vi "JKISM-Reuse Module.vi"(7 "Name(\"\" to use uuid)":string="Event JKISM") -> ()   [LabVIEW 2014]
uses:
  user.lib/_NEVSTOP/JKI State Machine++/_Support/JKISMQ/_Obtain JKISMQ.vi
  user.lib/_NEVSTOP/JKI State Machine++/_Support/FGV-BroadcastRegistry/Cache-Broadcast Registry Search Result.vi
  user.lib/_NEVSTOP/JKI State Machine++/AdvanceAPI/JKISM++ Register Status Change.vi
  user.lib/_NEVSTOP/JKI State Machine++/AdvanceAPI/JKISM++ Unregister Status Change.vi
  user.lib/_NEVSTOP/JKI State Machine++/_Support/JKISMQ/_Create Resp Queue.vi
  user.lib/_NEVSTOP/JKI State Machine++/_Support/JKISMQ/_Unlock JKISMQ.vi
  user.lib/_NEVSTOP/JKI State Machine++/_Support/JKISMQ/_Lock State JKISMQ.vi
  user.lib/_NEVSTOP/JKI State Machine++/_Support/JKISMQ/_Release JKISMQ.vi
  user.lib/_NEVSTOP/JKI State Machine++/AdvanceAPI/JKISM++ Make String Arguments Safe.vi
  user.lib/_NEVSTOP/JKI State Machine++/_Support/JKISMQ/_Input Name to JKISM Mode.vi
  user.lib/_NEVSTOP/JKI State Machine++/Utility/uuid.vi
  user.lib/_NEVSTOP/JKI State Machine++/_Support/KeyWords.vi
  user.lib/_NEVSTOP/JKI State Machine++/_Support/FGV-BroadcastRegistry/global-JKISMQ FGV Change Flag.vi
  user.lib/_NEVSTOP/JKI State Machine++/_Support/JKISMQ/_JKISMQFGV.vi
  user.lib/_NEVSTOP/JKI State Machine++/_Support/GlobalEvent/FGV-GlobalEventRef.vi
  user.lib/_NEVSTOP/JKI State Machine++/_Support/JKISMQ/_Dequeue JKISMQ.vi
  user.lib/_NEVSTOP/JKI State Machine++/_Support/JKISMQ/_Enqueue JKISMQ.vi
  user.lib/_NEVSTOP/JKI State Machine++/_Support/FGV-BroadcastRegistry/global-Broadcast Cache Change Flag.vi
  user.lib/_NEVSTOP/JKI State Machine++/_Support/FGV-BroadcastRegistry/FGV-BroadcastRegistry.vi
  user.lib/_NEVSTOP/JKI State Machine++/JKI State Machine++.lvlib
panel:
  in  "Stop":bool
  in  "Start":bool
  out "publish status":bool
  out "Random":dbl
  in  "Level":dbl=0.5 format="%#_13g"
  out "State History":string
  # ">"
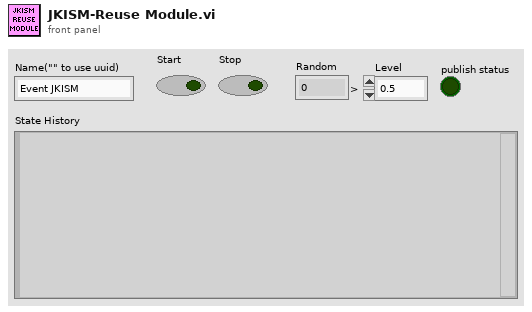
[diagram p1: front panel]
types:
  T1 = enum32{"Invalid", "Standard", "Closed", "Hidden", "Minimized", "Maximized"}
  T2 = enum32{"invalid app kind", "Development System", "Run Time System", "Student Edition", "Embedded LabVIEW", "Evaluation", "Custom"}
  T3 = cluster{"Core":cluster{"Current VI Reference":refnum<vi>, "Close Panel on Exit?":bool}, "Your Boolean data":bool, "Your string data":string}
  T4 = cluster{"Current VI Reference":refnum<vi>, "Close Panel on Exit?":bool}
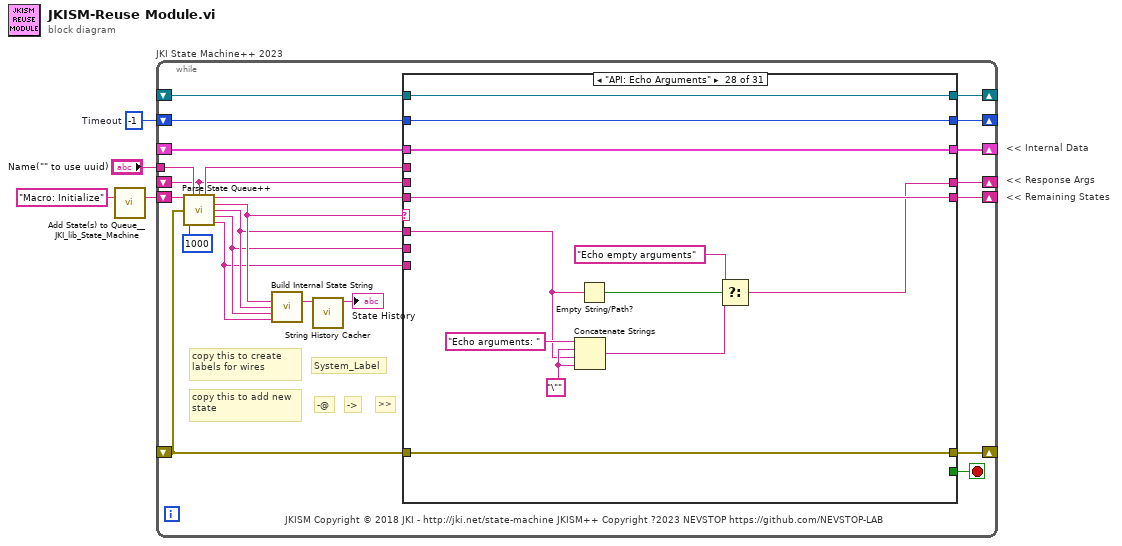
[diagram p0: block diagram]
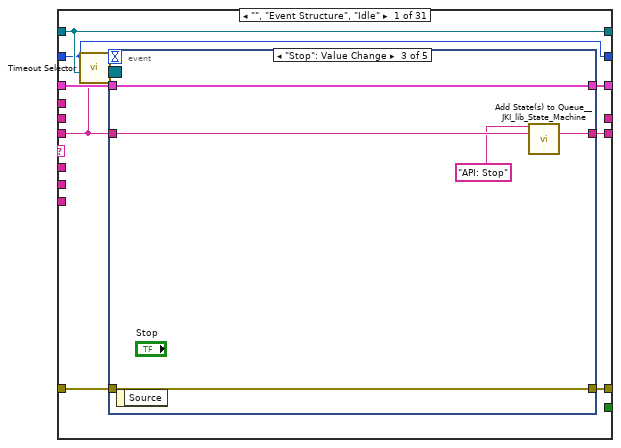
[diagram p2: hidden frame]
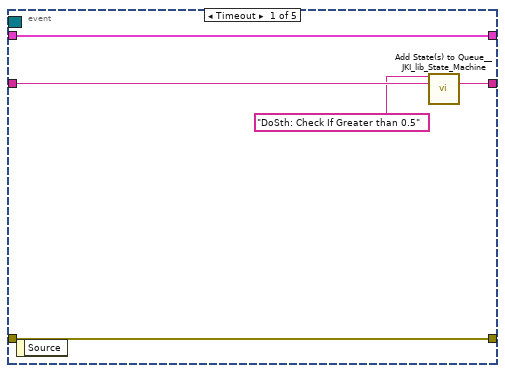
[diagram p3: hidden frame]
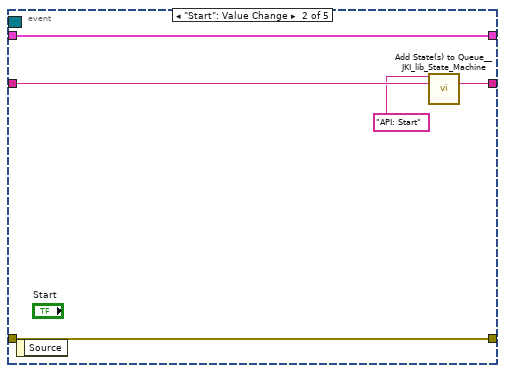
[diagram p4: hidden frame]
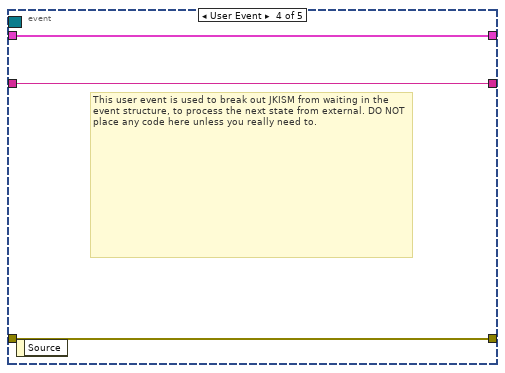
[diagram p5: hidden frame]
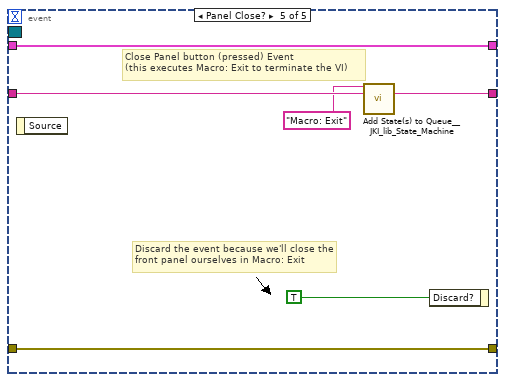
[diagram p6: hidden frame]
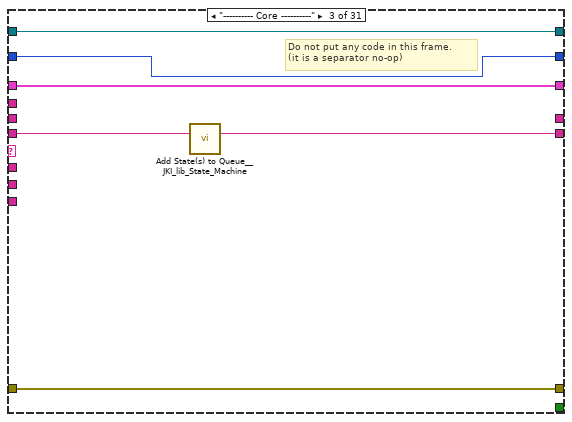
[diagram p8: hidden frame]
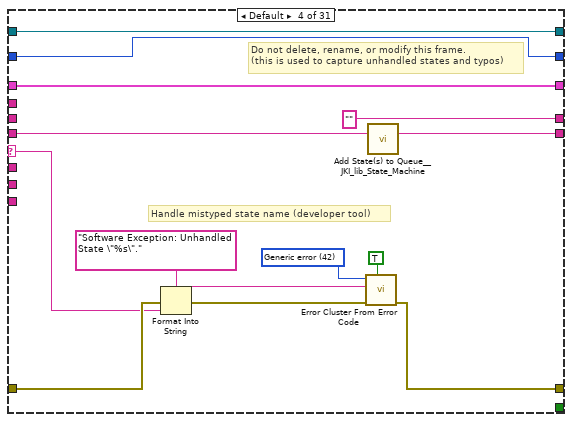
[diagram p9: hidden frame]
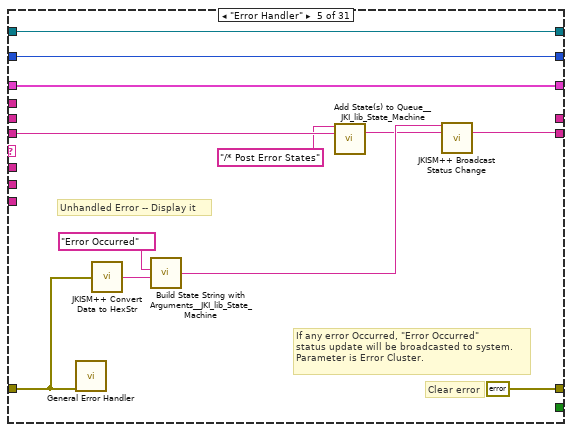
[diagram p10: hidden frame]
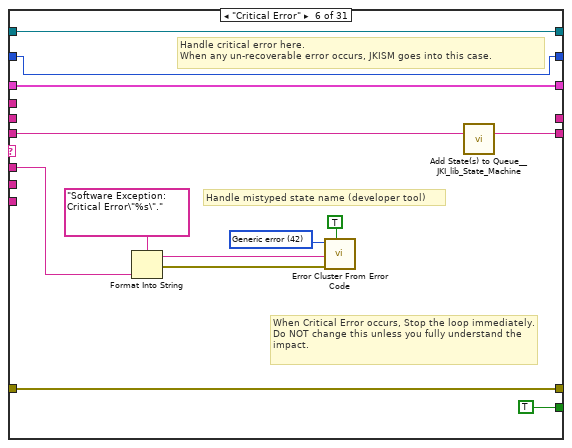
[diagram p11: hidden frame]
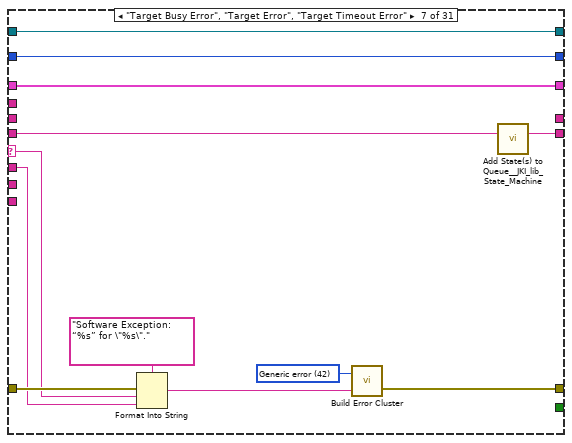
[diagram p12: hidden frame]
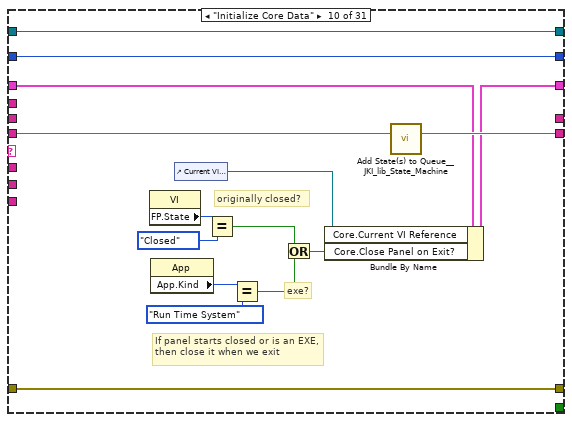
[diagram p15: hidden frame]
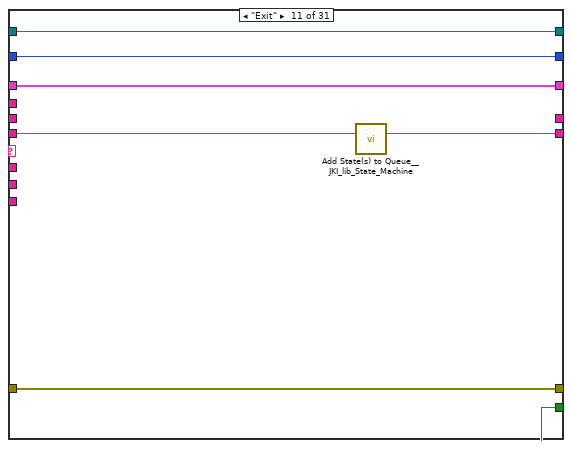
[diagram p16: hidden frame]
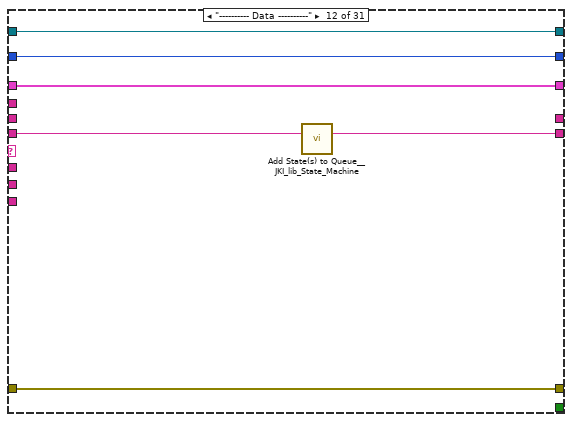
[diagram p17: hidden frame]
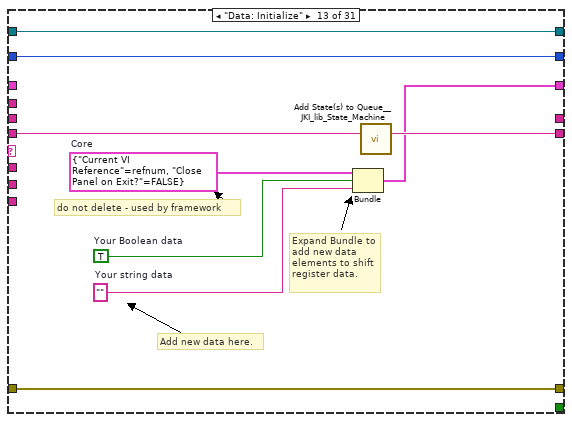
[diagram p18: hidden frame]
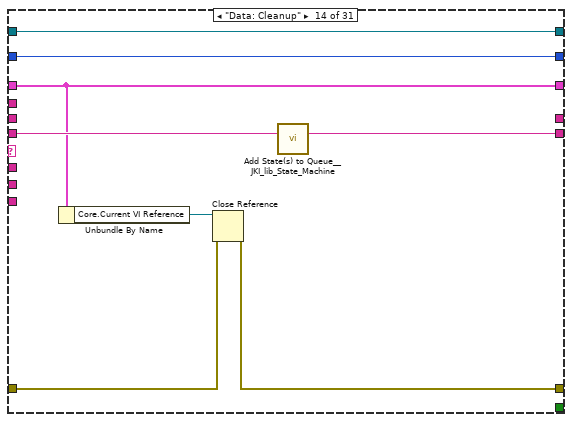
[diagram p19: hidden frame]
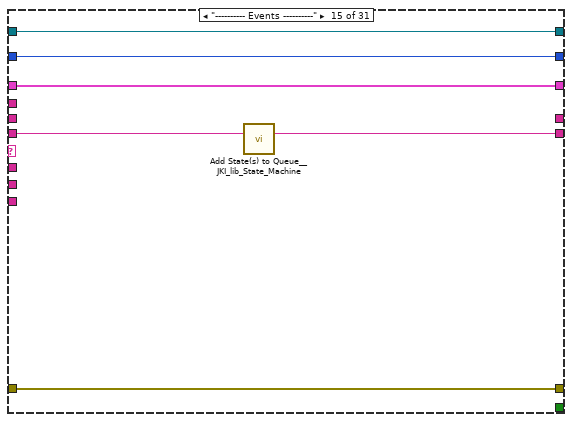
[diagram p20: hidden frame]
diagram:
  w1 = -1  # Timeout
  # "<< Internal Data"
  # "<< Response Args"
  # "<< Remaining States"
  n1 = call <vilib>:"Add State(s) to Queue__JKI_lib_State_Machine.vi"("State(s) in (\"\")"="Macro: Initialize") -> ("States Out"=w4:string)  [unwired: 14 in]
  n2 = while "JKI State Machine++ 2023" {
    shift-right: [w22] -> _
    shift-left: _ -> [w21]
    shift-right: [w25] -> _
    shift-left: _ -> [w20]
    shift-right: [w24] -> _
    shift-left: w4 -> [w26]
    tunnel: "Name(\"\" to use uuid)" -> [w15]
    shift-right: [w18] -> _
    shift-left: _ -> [w7]
    shift-right: [w17] -> _
    shift-left: _ -> [w16]
    shift-right: [w5] -> _
    shift-left: w1 -> [w6]
    stop <- w23 stop-if-true
    # "JKISM Copyright © 2018 JKI - http://jki.net/state-machine JKISM++ Copyright ?2023 NEVSTOP https://github.com/NEVSTOP-LAB"
    # "copy this to add new state"
    # ">>"
    # "->"
    # "-@"
    # "copy this to create labels for wires"
    # "System_Label"
    n3 = call "Parse State Queue++.vi"("State Queue"=w26, "Name(\"\" to use uuid)"=w15, "Response Arguments"=w7, "Error In (no error)"=w20, "Response Timeout(5000ms)"=1000 ("Response Timeout(1000ms)")) -> ("Name Used"=w8:string, "Remaining States"=w27:string, "Current State"=w12:string, "Arguments"=w11:string, "Argument - State"=w10:string, "From Who"=w9:string)  [unwired: 5 in]
    n4 = call "Build Internal State String.vi"("State"=w12, "Arguments (\"\")"=w11, "Arg-State (\"\")"=w10, "Source (\"\")"=w9) -> ("State with Arguments"=w13:string)  [unwired: 11 in]
    n5 = call "String History Cacher.vi"("String"=w13) -> ("String Cache"=→"State History":string)  [unwired: 10 in]
    n6 = case shown="\"API: Echo Arguments\"" w12 {
      selector: w12 -> [_ _ _ w75 _ _ w112 _ _ _ _ _ _ _ _ _ _ _ _ _ _ _ _ _ _ _ _ _ _ _ _]
      tunnel: w27 -> [w29 w64 w71 w79 w97 w108 w114 w126 w131 w147 w154 w160 w169 w177 w183 w190 w195 w202 w208 w216 w233 w304 w311 w323 w327 w335 w343 w355 w362 w371 w383]
      tunnel: w11 -> [_ _ _ _ _ w101 w113 _ _ _ _ _ _ _ _ _ _ _ _ w211 w227 _ _ _ _ _ _ w349 w359 _ _]
      tunnel: w21 -> [w35 w63 w68 w77 w95 w109 w116 w125 w130 w140 w152 w157 _ w172 w180 w189 w194 w199 w206 w214 w229 w301 w308 w320 w326 w334 w342 w354 w361 w368 w380]
      tunnel: [w34 w65 w69 w81 errorcluster {"status"=FALSE, "code"=0, "source"=""} ("error out") w110 w119 w127 w132 w144 w151 w158 w166 w173 w181 w185 w193 w200 w205 w212 w230 w302 w309 w321 w328 w336 w344 w356 w363 w369 w381] -> w25
      tunnel: w20 -> [w33 w65 w69 w80 w87 w110 w118 w127 w132 w144 w151 w158 w166 w174 w181 _ w196 w200 w205 w213 w231 w302 w309 w321 w328 w336 w344 w356 w363 w369 w381]
      tunnel: [w36 w64 w70 w78 w88 w107 w117 w126 w131 w146 w153 w159 w168 w176 w182 w190 w195 w201 w207 w215 w232 w303 w310 w322 w327 w335 w343 w355 w362 w370 w382] -> w24
      tunnel: [_ _ _ _ _ TRUE _ _ _ _ TRUE _ _ _ _ _ _ _ _ _ _ _ _ _ _ _ _ _ _ _ _] -> w23
      tunnel: [w32 w63 w68 w77 w95 w109 w116 w125 w130 w145 w152 w157 w167 w172 w180 w189 w194 w199 w206 w214 w229 w301 w308 w320 w326 w334 w342 w354 w361 w368 w380] -> w22
      tunnel: w6 -> [w28 w61 w66 w72 w86 w98 w111 w123 w128 w133 w148 w155 w161 w170 w178 w184 w191 w197 w203 w209 w225 w299 w305 w312 w324 _ _ w352 w357 w366 w372]
      tunnel: w9 -> [_ _ _ _ _ _ _ _ _ _ _ _ _ _ _ _ _ _ _ _ _ _ _ _ _ _ _ _ _ _ _]
      tunnel: w10 -> [_ _ _ _ _ _ _ _ _ _ _ _ _ _ _ _ _ _ _ _ _ _ _ _ _ _ _ _ _ _ _]
      tunnel: [_ _ _ "" _ _ _ _ _ _ _ _ _ _ _ _ _ _ _ _ _ _ _ _ _ w330 w338 w346 w358 _ _] -> w18
      tunnel: [w31 w62 w67 w73 w93 w99 w115 w124 w129 w134 w149 w156 w162 w171 w179 w188 w192 w198 w204 w210 w226 w300 w306 w313 w325 w333 w341 w353 w360 w367 w379] -> w17
      tunnel: w16 -> [w31 w62 w67 w73 w93 w99 w115 w124 w129 w134 w149 w156 w162 w171 w179 _ w192 w198 w204 w210 w226 w300 w306 w313 w325 w333 w341 w353 w360 w367 w379]
      tunnel: w8 -> [_ _ _ _ _ _ _ _ _ _ _ _ _ _ _ w187 _ _ _ _ _ _ _ _ _ w329 w337 _ _ _ _]
      tunnel: w7 -> [_ _ _ _ _ _ _ _ _ _ _ _ _ _ _ _ _ _ _ _ _ _ _ _ _ _ _ _ _ _ _]
      tunnel: [w28 w61 w66 w72 w86 w98 w111 w123 w128 w133 w148 w155 w161 w170 w178 w184 w191 w197 w203 w209 w225 w299 w305 w312 w324 1000 ("Timeout") -1 ("Timeout") w352 w357 w366 w372] -> w5
      frame "", "Event Structure", "Idle" {
        n7 = call "Timeout Selector.vi"("Remaining States"=w29, "Timeout Expected"=w28) -> ("Timeout"=w30:i32)  [unwired: 5 in]
        n8 = event shown="[2] \"Stop\": Value Change" {
          selector: w31 -> [_ _ _ _ _]
          dyn-events: _ -> [_ _ _ _ _]
          timeout: w30 -> [_ _ _ _ _]
          tunnel: w29 -> [w41 w46 w51 w53 w60]
          tunnel: [w40 w45 w50 w53 w59] -> w36
          tunnel: w35 -> [w38 w43 w48 w54 w57]
          tunnel: [w39 w44 w49 w52 w58] -> w34
          tunnel: w33 -> [w39 w44 w49 w52 w58]
          tunnel: [w38 w43 w48 w54 w57] -> w32
          event Timeout {
            n9 = event-data() -> ()  [unwired: 1 in, 1 out]
            n10 = call <vilib>:"Add State(s) to Queue__JKI_lib_State_Machine.vi"("State(s) in Front (\"\")"="DoSth: Check If Greater than 0.5" ("State(s) in Front (\"\")"), "State(s) in (\"\")"=w41) -> ("States Out"=w40:string)  [unwired: 13 in]
          }
          event "Start": Value Change {
            n11 = event-data() -> ()  [unwired: 1 in, 1 out]
            n12 = call <vilib>:"Add State(s) to Queue__JKI_lib_State_Machine.vi"("State(s) in Front (\"\")"="API: Start" ("State(s) in Front (\"\")"), "State(s) in (\"\")"=w46) -> ("States Out"=w45:string)  [unwired: 13 in]
          }
          event "Stop": Value Change {
            n13 = event-data() -> ()  [unwired: 1 in, 1 out]
            n14 = call <vilib>:"Add State(s) to Queue__JKI_lib_State_Machine.vi"("State(s) in Front (\"\")"="API: Stop" ("State(s) in Front (\"\")"), "State(s) in (\"\")"=w51) -> ("States Out"=w50:string)  [unwired: 13 in]
          }
          event User Event {
            # "This user event is used to break out JKISM from waiting in the event structure, to process the next state from external. DO NOT place any code here unless you really need to."
            n15 = event-data() -> ()  [unwired: 1 in, 1 out]
          }
          event Panel Close? {
            # "Discard the event because we'll close the front panel ourselves in Macro: Exit"
            # "Close Panel button (pressed) Event\n(this executes Macro: Exit to terminate the VI)"
            n16 = event-data() -> ()  [unwired: 1 in, 1 out]
            n17 = call <vilib>:"Add State(s) to Queue__JKI_lib_State_Machine.vi"("State(s) in Front (\"\")"="Macro: Exit", "State(s) in (\"\")"=w60) -> ("States Out"=w59:string)  [unwired: 13 in]
            n18 = event-data("Discard?"=TRUE) -> ()  [unwired: 1 in, 1 out]
          }
        }
      }
      frame "JKISM++ Documentation" {
        # "JKISM++ Documentation"
        # "State Syntax:\nStateCategory: State >> Argument -@ JKISMName\nStateCategory: State >> Argument -> JKISMName\n\nLine Terminator: Line feed"
        # "Commenting:\nTo add a comment use \"//\" or \"#\" and all text to the right will be ignored\nCommenting Example:\nUI: Initialize // This initializes the UI\n# This whole line is a comment\n// Another comment line"
      }
      frame "---------- Core ----------" {
        # "Do not put any code in this frame.\n(it is a separator no-op)"
        n19 = call <vilib>:"Add State(s) to Queue__JKI_lib_State_Machine.vi"("State(s) in (\"\")"=w71) -> ("States Out"=w70:string)  [unwired: 14 in]
      }
      frame Default {
        w84 = 42 items=["No error", "Argument error", "Memory is full", "Out of zone", "End of file", "File already open", "Generic file I/O error", "File not found", "File permission error", "Disk is full", "Duplicate path", "Too many files open", "System feature not enabled", "Resource file not found", "Cannot add resource", "Resource not found", "Image not found", "Image memory error", "Pen does not exist", "Config type invalid", "Config token not found", "Config parse error", "Config memory error", "Bad external code format", "Bad external code offset", "External code not present", "Null window", "Destroy window error", "Null menu", "Print aborted", "Bad print record", "Print driver error", "Windows error during printing", "Memory error during printing", "Print dialog error", "Generic print error", "Invalid device refnum", "Device not found", "Device parameter error", "Device unit error", "Cannot open device", "Device call aborted", "Generic error", "Cancelled by user", "Object ID too low", "Object ID too high", "Object not in heap", "Unknown heap", "Unknown object (invalid DefProc)", "Unknown object (DefProc not in table)", "Message out of range", "Invalid (null) method", "Unknown message", "Manager call not supported", "Bad address", "Network operation in progress", "Network operation timed out", "Connection is busy", "Network attribute not supported", "Network error", "Address in use", "System out of memory", "Connection aborted", "Connection refused", "Not connected", "Already connected", "Connection closed", "Initialization error (interapplication manager)", "Bad occurrence", "Wait on unbound occurrence handler", "Occurrence queue overflow", "Datalog type conflict", "Unused", "Unrecognized type (interapplication manager)", "Memory corrupt", "Failed to make temporary DLL", "Old CIN version", "Drag socket not found", "Failed to load drop-object", "Failed to register OLE object", "Failed to release OLE object", "Format specifier type mismatch", "Unknown format specifier", "Too few format specifiers", "Too many format specifiers", "Scan failed", "Newer CIN version", "Error converting to variant", "Runtime menu error", "Password tampered", "Variant attribute not found", "Incompatible variant data type", "Event data is not available", "Event Store is not present", "Occurrence is not found", "Event Queue is not created", "Event info is not available", "Refnum passed is NULL", "Error retrieving Class GUID", "Error retrieving CoClass GUID", "Error retrieving TypeLib GUID.", "Bad built application magic bytes.", "Specific driver is different from the specific driver associated with the Logical Name.", "There is no session opened to the class driver.", "Max Error", "MAX - Error with config objects", "MAX - Error loading configuration", "MAX - Group not supported"]
        # "Do not delete, rename, or modify this frame.\n(this is used to capture unhandled states and typos)"
        # "Handle mistyped state name (developer tool)"
        n20 = Format Into String(format string="Software Exception: Unhandled State \"%s\"." ("message"), error in=w80, w75) -> (resulting string=w83:string, error out=w82:errorcluster)  [unwired: 1 in]
        n21 = call <vilib>:"Error Cluster From Error Code.vi"("show call chain? (False)"=TRUE, "error in (no error)"=w82, "error message (\"\")"=w83, "error code (0)"=w84) -> ("error out"=w81:errorcluster)  [unwired: 5 in]
        n22 = call <vilib>:"Add State(s) to Queue__JKI_lib_State_Machine.vi"("State(s) in (\"\")"=w79) -> ("States Out"=w78:string)  [unwired: 14 in]
      }
      frame "Error Handler" {
        # "If any error Occurred, \"Error Occurred\" \nstatus update will be broadcasted to system.\nParameter is Error Cluster."
        # "Unhandled Error -- Display it"
        # "Clear error"
        n23 = call <vilib>:"General Error Handler.vi"("error in (no error)"=w87) -> ()  [unwired: 10 in, 5 out]
        n24 = call "JKISM++ Convert Data to HexStr.vi"("Variant"=w87) -> ("HEX String (0-9,A-F)"=w91:string)  [unwired: 8 in]
        n25 = call <vilib>:"Build State String with Arguments__JKI_lib_State_Machine.vi"("Arguments (\"\")"=w91, "State"="Error Occurred" ("Status with Arguments")) -> ("State with Arguments"=w90:string)  [unwired: 4 in]
        n26 = call <vilib>:"Add State(s) to Queue__JKI_lib_State_Machine.vi"("State(s) in Front (\"\")"="/* Post Error States", "State(s) in (\"\")"=w97) -> ("States Out"=w89:string)  [unwired: 13 in]
        n27 = call "JKISM++ Broadcast Status Change.vi"("Status with Arguments"=w90, "State Queue"=w89) -> ("Remaining States"=w88:string)  [unwired: 13 in]
      }
      frame "Critical Error" {
        w105 = 42 items=["No error", "Argument error", "Memory is full", "Out of zone", "End of file", "File already open", "Generic file I/O error", "File not found", "File permission error", "Disk is full", "Duplicate path", "Too many files open", "System feature not enabled", "Resource file not found", "Cannot add resource", "Resource not found", "Image not found", "Image memory error", "Pen does not exist", "Config type invalid", "Config token not found", "Config parse error", "Config memory error", "Bad external code format", "Bad external code offset", "External code not present", "Null window", "Destroy window error", "Null menu", "Print aborted", "Bad print record", "Print driver error", "Windows error during printing", "Memory error during printing", "Print dialog error", "Generic print error", "Invalid device refnum", "Device not found", "Device parameter error", "Device unit error", "Cannot open device", "Device call aborted", "Generic error", "Cancelled by user", "Object ID too low", "Object ID too high", "Object not in heap", "Unknown heap", "Unknown object (invalid DefProc)", "Unknown object (DefProc not in table)", "Message out of range", "Invalid (null) method", "Unknown message", "Manager call not supported", "Bad address", "Network operation in progress", "Network operation timed out", "Connection is busy", "Network attribute not supported", "Network error", "Address in use", "System out of memory", "Connection aborted", "Connection refused", "Not connected", "Already connected", "Connection closed", "Initialization error (interapplication manager)", "Bad occurrence", "Wait on unbound occurrence handler", "Occurrence queue overflow", "Datalog type conflict", "Unused", "Unrecognized type (interapplication manager)", "Memory corrupt", "Failed to make temporary DLL", "Old CIN version", "Drag socket not found", "Failed to load drop-object", "Failed to register OLE object", "Failed to release OLE object", "Format specifier type mismatch", "Unknown format specifier", "Too few format specifiers", "Too many format specifiers", "Scan failed", "Newer CIN version", "Error converting to variant", "Runtime menu error", "Password tampered", "Variant attribute not found", "Incompatible variant data type", "Event data is not available", "Event Store is not present", "Occurrence is not found", "Event Queue is not created", "Event info is not available", "Refnum passed is NULL", "Error retrieving Class GUID", "Error retrieving CoClass GUID", "Error retrieving TypeLib GUID.", "Bad built application magic bytes.", "Specific driver is different from the specific driver associated with the Logical Name.", "There is no session opened to the class driver.", "Max Error", "MAX - Error with config objects", "MAX - Error loading configuration", "MAX - Group not supported"]
        # "Handle critical error here.\nWhen any un-recoverable error occurs, JKISM goes into this case."
        # "When Critical Error occurs, Stop the loop immediately. Do NOT change this unless you fully understand the impact."
        # "Handle mistyped state name (developer tool)"
        n28 = Format Into String(format string="Software Exception: Critical Error\"%s\"." ("message"), w101) -> (resulting string=w104:string, error out=w103:errorcluster)  [unwired: 2 in]
        n29 = call <vilib>:"Error Cluster From Error Code.vi"("show call chain? (False)"=TRUE, "error in (no error)"=w103, "error message (\"\")"=w104, "error code (0)"=w105) -> ()  [unwired: 5 in, 1 out]
        n30 = call <vilib>:"Add State(s) to Queue__JKI_lib_State_Machine.vi"("State(s) in (\"\")"=w108) -> ("States Out"=w107:string)  [unwired: 14 in]
      }
      frame "Target Busy Error", "Target Error", "Target Timeout Error" {
        w121 = 42 items=["No error", "Argument error", "Memory is full", "Out of zone", "End of file", "File already open", "Generic file I/O error", "File not found", "File permission error", "Disk is full", "Duplicate path", "Too many files open", "System feature not enabled", "Resource file not found", "Cannot add resource", "Resource not found", "Image not found", "Image memory error", "Pen does not exist", "Config type invalid", "Config token not found", "Config parse error", "Config memory error", "Bad external code format", "Bad external code offset", "External code not present", "Null window", "Destroy window error", "Null menu", "Print aborted", "Bad print record", "Print driver error", "Windows error during printing", "Memory error during printing", "Print dialog error", "Generic print error", "Invalid device refnum", "Device not found", "Device parameter error", "Device unit error", "Cannot open device", "Device call aborted", "Generic error", "Cancelled by user", "Object ID too low", "Object ID too high", "Object not in heap", "Unknown heap", "Unknown object (invalid DefProc)", "Unknown object (DefProc not in table)", "Message out of range", "Invalid (null) method", "Unknown message", "Manager call not supported", "Bad address", "Network operation in progress", "Network operation timed out", "Connection is busy", "Network attribute not supported", "Network error", "Address in use", "System out of memory", "Connection aborted", "Connection refused", "Not connected", "Already connected", "Connection closed", "Initialization error (interapplication manager)", "Bad occurrence", "Wait on unbound occurrence handler", "Occurrence queue overflow", "Datalog type conflict", "Unused", "Unrecognized type (interapplication manager)", "Memory corrupt", "Failed to make temporary DLL", "Old CIN version", "Drag socket not found", "Failed to load drop-object", "Failed to register OLE object", "Failed to release OLE object", "Format specifier type mismatch", "Unknown format specifier", "Too few format specifiers", "Too many format specifiers", "Scan failed", "Newer CIN version", "Error converting to variant", "Runtime menu error", "Password tampered", "Variant attribute not found", "Incompatible variant data type", "Event data is not available", "Event Store is not present", "Occurrence is not found", "Event Queue is not created", "Event info is not available", "Refnum passed is NULL", "Error retrieving Class GUID", "Error retrieving CoClass GUID", "Error retrieving TypeLib GUID.", "Bad built application magic bytes.", "Specific driver is different from the specific driver associated with the Logical Name.", "There is no session opened to the class driver.", "Max Error", "MAX - Error with config objects", "MAX - Error loading configuration", "MAX - Group not supported"]
        n31 = Format Into String(format string="Software Exception: “%s” for \"%s\"." ("message"), error in=w118, w112, w113) -> (resulting string=w120:string)  [unwired: 1 in, 1 out]
        n32 = call "Build Error Cluster.vi"("String to Prepend to source (\"\")"=w120, "code"=w121) -> ("error out"=w119:errorcluster)
        n33 = call <vilib>:"Add State(s) to Queue__JKI_lib_State_Machine.vi"("State(s) in (\"\")"=w114) -> ("States Out"=w117:string)  [unwired: 14 in]
      }
      frame "Async Response", "Response" {
        # "Handle Async-call Response (\"Async Response\" for ->)"
        # "Handle Sync-call Response (\"Response\" for @)"
        # "After Message is executed, JKISM+ goes to this state for receive the response. \n    For Async Message(->), \"Async Response\" is used. This JKISM will goes to \"Async Message Posted\" immediately and receive the \"Async Response\" after the callee finishes the message.\n    For Sync Message(@),  This JKISM will wait until the message is done and immediately goes to \"Response\""
      }
      frame "Async Message Posted" {
        # "Handle post action for async message (->)."
        # "After Async Message is posted (->), JKISM+ goes to this state for post-action. You can use Argument - State to tell which Async Message is called."
      }
      frame "Initialize Core Data" {
        # "originally closed?"
        # "exe?"
        # "If panel starts closed or is an EXE, then close it when we exit"
        n34 = property class="VI"() -> ("FP.State"=w137:T1)  [unwired: 2 in, 2 out]
        n35 = property class="App"() -> ("App.Kind"=w143:T2)  [unwired: 2 in, 2 out]
        n36 = control-ref of="Current VI Reference"() -> (w138:refnum<vi>)
        n37 = Equal?(x=w137, y=T1."Closed" ("Front Panel Window:State")) -> (x = y?=w135:bool)
        n38 = Equal?(x=w143, y=T2."Run Time System" ("Application:Kind")) -> (x = y?=w141:bool)
        n39 = Or(x=w135, y=w141) -> (x .or. y?=w139:bool)
        n40 = Bundle By Name(cluster=w140, "Core.Current VI Reference"=w138, "Core.Close Panel on Exit?"=w139) -> (w145:T3)
        n41 = call <vilib>:"Add State(s) to Queue__JKI_lib_State_Machine.vi"("State(s) in (\"\")"=w147) -> ("States Out"=w146:string)  [unwired: 14 in]
      }
      frame "Exit" {
        n42 = call <vilib>:"Add State(s) to Queue__JKI_lib_State_Machine.vi"("State(s) in (\"\")"=w154) -> ("States Out"=w153:string)  [unwired: 14 in]
      }
      frame "---------- Data ----------" {
        n43 = call <vilib>:"Add State(s) to Queue__JKI_lib_State_Machine.vi"("State(s) in (\"\")"=w160) -> ("States Out"=w159:string)  [unwired: 14 in]
      }
      frame "Data: Initialize" {
        w163 = T4 {"Current VI Reference"=refnum, "Close Panel on Exit?"=FALSE}  # Core
        w165 = TRUE  # Your Boolean data
        w164 = ""  # Your string data
        # "do not delete - used by framework"
        # "Expand Bundle to add new data elements to shift register data."
        # "Add new data here."
        n44 = Bundle("Core"=w163, "Your Boolean data"=w165, "Your string data"=w164) -> (w167:T3)  [unwired: 1 in]
        n45 = call <vilib>:"Add State(s) to Queue__JKI_lib_State_Machine.vi"("State(s) in (\"\")"=w169) -> ("States Out"=w168:string)  [unwired: 14 in]
      }
      frame "Data: Cleanup" {
        n46 = Unbundle By Name(w172) -> ("Core.Current VI Reference"=w175:refnum<vi>)
        n47 = Close Reference(reference=w175, error in (no error)=w174) -> (error out=w173:errorcluster)
        n48 = call <vilib>:"Add State(s) to Queue__JKI_lib_State_Machine.vi"("State(s) in (\"\")"=w177) -> ("States Out"=w176:string)  [unwired: 14 in]
      }
      frame "---------- Events ----------" {
        n49 = call <vilib>:"Add State(s) to Queue__JKI_lib_State_Machine.vi"("State(s) in (\"\")"=w183) -> ("States Out"=w182:string)  [unwired: 14 in]
      }
      frame "Events: Register" {
        # "Register message event to break Waiting in Event structure."
        n50 = call "JKISM++ Get New State Notifier Event.vi"("Name(\"\" to use uuid) in"=w187) -> ("Error out"=w185:errorcluster, "New State Notifier Event"=w186:refnum<user-event>)  [unwired: 9 in]
        n51 = register-events(w186) -> (reference out=w188:refnum<event-registration>)  [unwired: 2 in, 1 out]
      }
      frame "Events: Unregister" {
        n52 = Unregister For Events(event registration refnum=w192, error in=w196) -> (error out=w193:errorcluster)
      }
      frame "---------- UI ----------" {
        n53 = call <vilib>:"Add State(s) to Queue__JKI_lib_State_Machine.vi"("State(s) in (\"\")"=w202) -> ("States Out"=w201:string)  [unwired: 14 in]
      }
      frame "UI: Initialize" {
        n54 = call <vilib>:"Add State(s) to Queue__JKI_lib_State_Machine.vi"("State(s) in (\"\")"=w208) -> ("States Out"=w207:string)  [unwired: 14 in]
      }
      frame "UI: Cursor Set" {
        # "Argument"
        n55 = disable-structure shown="Default" {
          disable-tunnel: w213 -> [w219 w224]
          disable-tunnel: [w218 w224] -> w212
          disable-tunnel: w211 -> [w217 _]
          frame condition #0 (active) {
            n56 = case shown="\"Idle\", Default" w217 {
              tunnel: w219 -> [w221 w223]
              tunnel: [w220 w222] -> w218
              frame "Idle", Default {
                n57 = call <vilib>:"Unset Busy.vi"("error in (no error)"=w221) -> ("error out"=w220:errorcluster)  [unwired: 10 in]
              }
              frame "Busy" {
                n58 = call <vilib>:"Set Busy.vi"("error in (no error)"=w223) -> ("error out"=w222:errorcluster)  [unwired: 9 in, 1 out]
              }
            }
          }
          frame condition #1 {
          }
        }
        n59 = call <vilib>:"Add State(s) to Queue__JKI_lib_State_Machine.vi"("State(s) in (\"\")"=w216) -> ("States Out"=w215:string)  [unwired: 14 in]
      }
      frame "UI: Front Panel State" {
        # "Argument"
        n60 = Unbundle By Name(w229) -> ("Core.Current VI Reference"=w228:refnum<vi>)
        n61 = call <vilib>:"Add State(s) to Queue__JKI_lib_State_Machine.vi"("State(s) in (\"\")"=w233) -> ("States Out"=w232:string)  [unwired: 14 in]
        n62 = case shown="\"Close\", \"Closed\"" w227 {
          tunnel: w231 -> [w239 w254 w265 w278 w291]
          tunnel: [w241 w255 w267 w280 w293] -> w230
          tunnel: w228 -> [w240 w252 w266 w279 w292]
          frame "Open", "Standard", Default {
            w234 = T1."Standard" ("State")
            n63 = property class="VI"(reference=w240, error in=w239) -> (reference out=w237:refnum<vi>, error out=w238:errorcluster, "FP.State"=w236:T1)
            n64 = Not Equal?(x=w236, y=w234) -> (x != y?=w235:bool)
            n65 = case shown="True" w235 {
              tunnel: [w245 w247] -> w241
              tunnel: w238 -> [w244 w247]
              tunnel: w237 -> [w243 _]
              tunnel: w234 -> [w242 _]
              frame True {
                n66 = invoke class="VI" method="FP.Open"(reference=w243, error in=w244, "Activate"=TRUE, "State"=w242) -> (error out=w245:errorcluster)  [unwired: 1 in, 4 out]
              }
              frame False {
              }
            }
          }
          frame "Close", "Closed" {
            n67 = property class="VI"(reference=w252, error in=w254) -> (reference out=w251:refnum<vi>, error out=w253:errorcluster, "FP.State"=w249:T1)
            n68 = Not Equal?(x=w249, y=T1."Closed" ("Front Panel Window:State")) -> (x != y?=w248:bool)
            n69 = case shown="True" w248 {
              tunnel: [w256 w259] -> w255
              tunnel: w253 -> [w256 w258]
              tunnel: w251 -> [_ w257]
              frame False {
              }
              frame True {
                n70 = invoke class="VI" method="FP.Close"(reference=w257, error in=w258) -> (error out=w259:errorcluster)  [unwired: 1 in, 2 out]
              }
            }
          }
          frame "Hidden", "Hide" {
            w260 = T1."Hidden" ("State")
            n71 = property class="VI"(reference=w266, error in=w265) -> (reference out=w263:refnum<vi>, error out=w264:errorcluster, "FP.State"=w262:T1)
            n72 = Not Equal?(x=w262, y=w260) -> (x != y?=w261:bool)
            n73 = case shown="True" w261 {
              tunnel: [w271 w272] -> w267
              tunnel: w264 -> [w270 w272]
              tunnel: w263 -> [w269 _]
              tunnel: w260 -> [w268 _]
              frame True {
                n74 = invoke class="VI" method="FP.Open"(reference=w269, error in=w270, "State"=w268) -> (error out=w271:errorcluster)  [unwired: 2 in, 4 out]
              }
              frame False {
              }
            }
          }
          frame "Minimize", "Minimized" {
            w273 = T1."Minimized" ("State")
            n75 = property class="VI"(reference=w279, error in=w278) -> (reference out=w276:refnum<vi>, error out=w277:errorcluster, "FP.State"=w275:T1)
            n76 = Not Equal?(x=w275, y=w273) -> (x != y?=w274:bool)
            n77 = case shown="True" w274 {
              tunnel: [w284 w285] -> w280
              tunnel: w277 -> [w283 w285]
              tunnel: w276 -> [w282 _]
              tunnel: w273 -> [w281 _]
              frame True {
                n78 = invoke class="VI" method="FP.Open"(reference=w282, error in=w283, "State"=w281) -> (error out=w284:errorcluster)  [unwired: 2 in, 4 out]
              }
              frame False {
              }
            }
          }
          frame "Maximize", "Maximized" {
            w286 = T1."Maximized" ("State")
            n79 = property class="VI"(reference=w292, error in=w291) -> (reference out=w289:refnum<vi>, error out=w290:errorcluster, "FP.State"=w288:T1)
            n80 = Not Equal?(x=w288, y=w286) -> (x != y?=w287:bool)
            n81 = case shown="True" w287 {
              tunnel: [w297 w298] -> w293
              tunnel: w290 -> [w296 w298]
              tunnel: w289 -> [w295 _]
              tunnel: w286 -> [w294 _]
              frame True {
                n82 = invoke class="VI" method="FP.Open"(reference=w295, error in=w296, "State"=w294) -> (error out=w297:errorcluster)  [unwired: 2 in, 4 out]
              }
              frame False {
              }
            }
          }
        }
      }
      frame "---------- Macro ----------" {
        n83 = call <vilib>:"Add State(s) to Queue__JKI_lib_State_Machine.vi"("State(s) in (\"\")"=w304) -> ("States Out"=w303:string)  [unwired: 14 in]
      }
      frame "Macro: Initialize" {
        w307 = "Data: Initialize\nInitialize Core Data\nEvents: Register\nUI: Initialize\nUI: Front Panel State >> Open"  # Data: Initialize Initialize Core Data Events: Register UI: Initialize UI: Front Panel State >> Open
        n84 = call <vilib>:"Add State(s) to Queue__JKI_lib_State_Machine.vi"("State(s) in Front (\"\")"=w307, "State(s) in (\"\")"=w311) -> ("States Out"=w310:string)  [unwired: 13 in]
      }
      frame "Macro: Exit" {
        n85 = Unbundle By Name(w320) -> ("Core.Close Panel on Exit?"=w319:bool)
        n86 = Select(t="UI: Front Panel State >> Close", s=w319, f="") -> (s? t:f=w316:string)
        n87 = call <vilib>:"Add State(s) to Queue__JKI_lib_State_Machine.vi"("State(s) in (\"\")"=w316, "State(s) at Back (\"\")"="Data: Cleanup\nEvents: Unregister\nExit") -> ("States Out"=w314:string)  [unwired: 13 in]
        n88 = call <vilib>:"Add State(s) to Queue__JKI_lib_State_Machine.vi"("State(s) in Front (\"\")"=w314, "State(s) in (\"\")"=w323) -> ("States Out"=w322:string)  [unwired: 13 in]
      }
      frame "---------- API ----------" {
      }
      frame "API: Start" {
        n89 = Concatenate Strings(w329, " Started") -> (w330:string)
      }
      frame "API: Stop" {
        n90 = Concatenate Strings(w337, " Stopped") -> (w338:string)
      }
      frame "API: Echo Arguments" {
        w350 = "\"" ("string")
        n91 = Concatenate Strings("Echo arguments: " ("string"), w350, w349, w350) -> (w347:string)
        n92 = Empty String/Path?(string/path=w349) -> (empty?=w348:bool)
        n93 = Select(t="Echo empty arguments" ("string"), s=w348, f=w347) -> (s? t:f=w346:string)
      }
      frame "API: Echo xxx" {
        # "unpack HexStr  to Variant\nif complex parameter is needed."
        n94 = call "JKISM++ Convert HexStr to Data.vi"("HEX String"=w359) -> ()  [unwired: 7 in, 2 out]
        n95 = disable-structure shown="Disabled" {
          disable-tunnel: [w364 "API2 Response"] -> w358
          frame Disabled {
            # "pack variant to hexstr \nif complex response is needed."
            # "complex Response"
            n96 = call "JKISM++ Convert Data to HexStr.vi"() -> ("HEX String (0-9,A-F)"=w364:string)  [unwired: 9 in]
          }
          frame Enabled {
          }
        }
      }
      frame "---------- DoSth ----------" {
        n97 = call <vilib>:"Add State(s) to Queue__JKI_lib_State_Machine.vi"("State(s) in (\"\")"=w371) -> ("States Out"=w370:string)  [unwired: 14 in]
      }
      frame "DoSth: Check If Greater than 0.5" {
        n98 = Random Number (0-1)() -> (number: 0 to 1=w376:dbl)
        "Random" <- w376
        n99 = Greater?(x=w376, y="Level") -> (0:w373:bool)
        "publish status" <- w373
        n100 = Format Into String(w376) -> (resulting string=w374:string)  [unwired: 3 in, 1 out]
        n101 = call <vilib>:"Build State String with Arguments__JKI_lib_State_Machine.vi"("Arguments (\"\")"=w374, "State"="Status Changed") -> ("State with Arguments"=w377:string)  [unwired: 4 in]
        n102 = call "JKISM++ Broadcast Status Change.vi"("Status with Arguments"=w377, "State Queue"=w383, "Broadcast(T)"=w373) -> ("Remaining States"=w382:string)  [unwired: 12 in]
      }
    }
  }
